vi "AssignFileChannels.vi"(10 "dataLoopCounter":dbl, 11 "dataTime_s":dbl) -> (3 "fileContent":T1)   [LabVIEW 2018]
uses:
  Clusters/FileDataChannel.ctl
  Clusters/IOSignals.ctl
  Clusters/ArrayPairs.ctl
  Clusters/SwapArrayCluster.ctl
  Clusters/GenCtrl.ctl
  Clusters/GenMode.ctl
  Clusters/PitchCtrl.ctl
  Clusters/BladePitchMode.ctl
  Clusters/RoscoParams.ctl
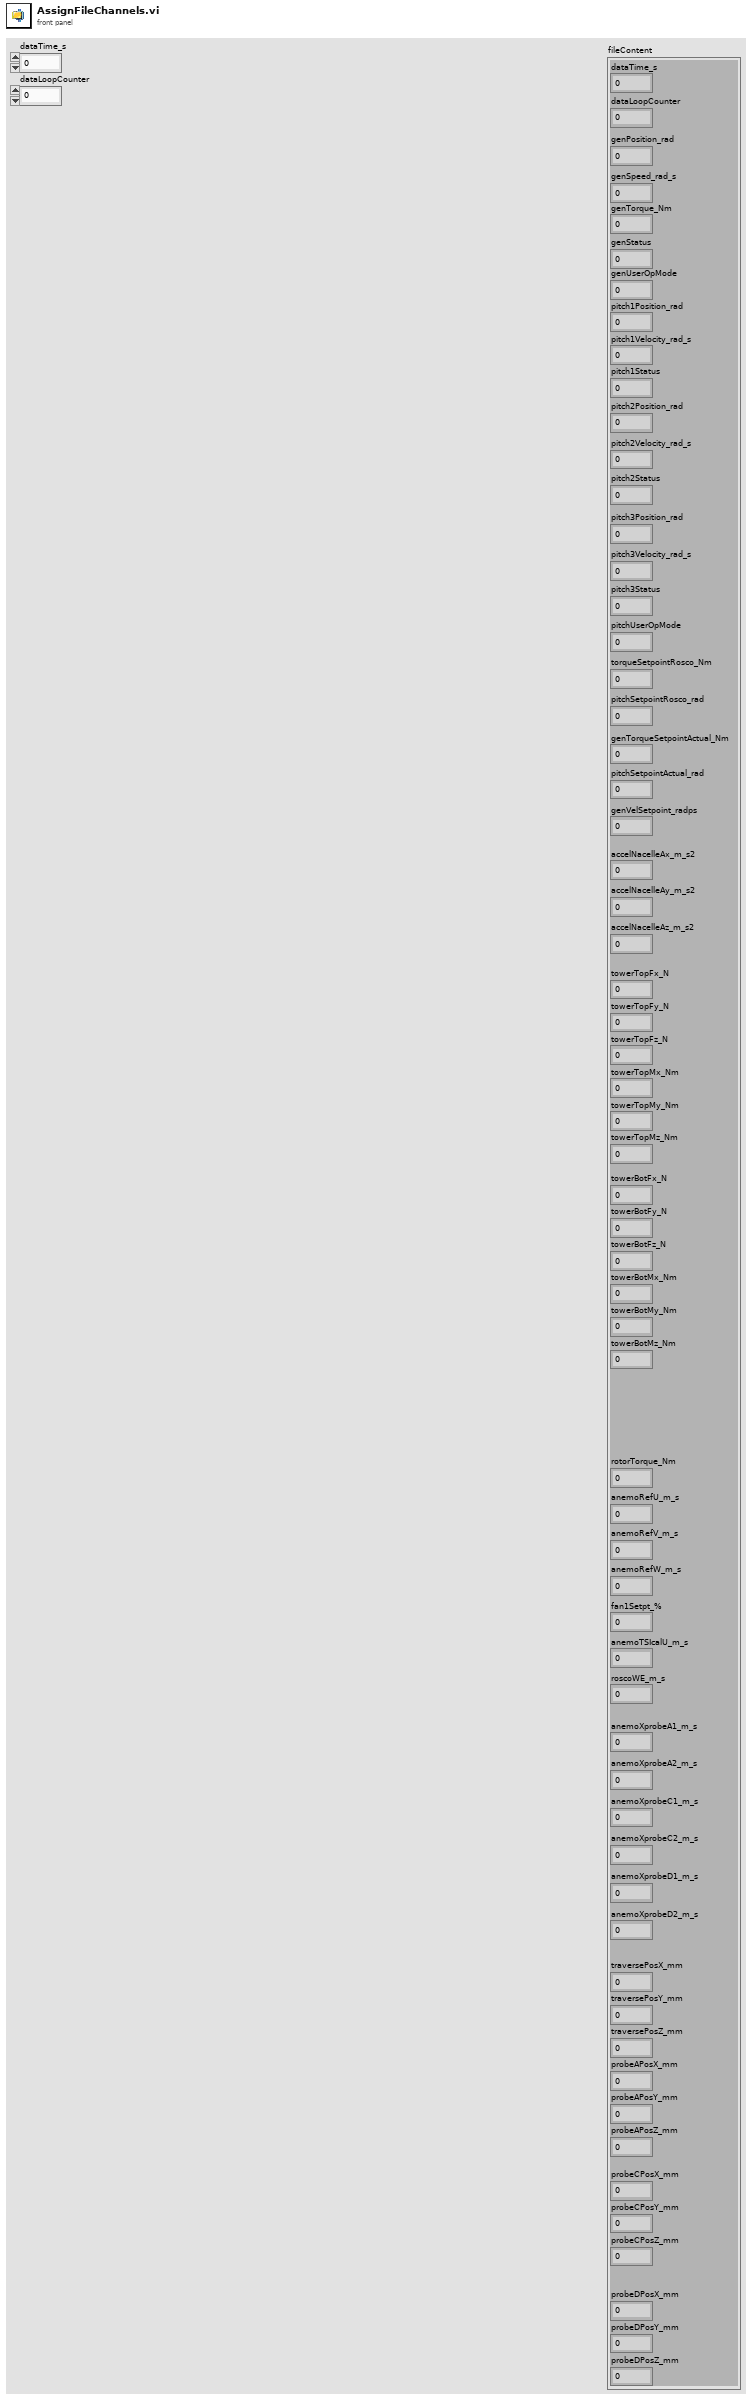
[diagram p1: front panel]
types:
  T1 = typedef "FileDataChannel.ctl" = cluster{"dataTime_s":dbl, "dataLoopCounter":dbl, "anemoRefU_m_s":dbl, "anemoRefV_m_s":dbl, "anemoRefW_m_s":dbl, "rotorTorque_Nm":dbl, "towerTopFx_N":dbl, "towerTopFy_N":dbl, "accelNacelleAx_m_s2":dbl, "accelNacelleAy_m_s2":dbl, "accelNacelleAz_m_s2":dbl, "genSpeed_rad_s":dbl, "genTorque_Nm":dbl, "genStatus":dbl, "pitch1Position_rad":dbl, "pitch1Velocity_rad_s":dbl, "pitch1Status":dbl, "pitch2Position_rad":dbl, "pitch2Velocity_rad_s":dbl, "pitch2Status":dbl, "pitch3Position_rad":dbl, "pitch3Velocity_rad_s":dbl, "pitch3Status":dbl, "genUserOpMode":dbl, "pitchUserOpMode":dbl, "torqueSetpointRosco_Nm":dbl, "pitchSetpointRosco_rad":dbl, "fan1Setpt_%":dbl, "genTorqueSetpointActual_Nm":dbl, "pitchSetpointActual_rad":dbl, "genVelSetpoint_radps":dbl, "genPosition_rad":dbl, "towerTopFz_N":dbl, "towerTopMx_Nm":dbl, "towerTopMy_Nm":dbl, "towerTopMz_Nm":dbl, "towerBotFx_N":dbl, "towerBotFy_N":dbl, "towerBotFz_N":dbl, "towerBotMx_Nm":dbl, "towerBotMy_Nm":dbl, "towerBotMz_Nm":dbl, "anemoTSIcalU_m_s":dbl, "roscoWE_m_s":dbl, "anemoXprobeA1_m_s":dbl, "anemoXprobeA2_m_s":dbl, "anemoXprobeC1_m_s":dbl, "anemoXprobeC2_m_s":dbl, "anemoXprobeD1_m_s":dbl, "anemoXprobeD2_m_s":dbl, "traversePosX_mm":dbl, "traversePosY_mm":dbl, "traversePosZ_mm":dbl, "probeAPosX_mm":dbl, "probeAPosY_mm":dbl, "probeAPosZ_mm":dbl, "probeCPosX_mm":dbl, "probeCPosY_mm":dbl, "probeCPosZ_mm":dbl, "probeDPosX_mm":dbl, "probeDPosY_mm":dbl, "probeDPosZ_mm":dbl}
  T2 = typedef "IOSignals.ctl" = cluster{"mainGenPosition (rad)":dbl, "mainGenVelocity (rad/s)":dbl, "motorCurrentTorq (Nm)":dbl, "mainGenStatus":u16, "pitch1Status":u16, "pitch1Position (rad)":dbl, "pitch1Velocity (rad/s)":dbl, "pitch1HomeFlag":bool, "pitch2Status":u16, "pitch2Position (rad)":dbl, "pitch2Velocity (rad/s)":dbl, "pitch2HomeFlag":bool, "pitch3Status":u16, "pitch3Position (rad)":dbl, "pitch3Velocity (rad/s)":dbl, "pitch3HomeFlag":bool, "torqueSensor (Nm)":dbl, "nacelleAccX (m/s2)":dbl, "nacelleAccY (m/s2)":dbl, "nacelleAccZ (m/s2)":dbl, "atiTowerTopFx_N":dbl, "atiTowerTopFy_N":dbl, "atiTowerTopFz_N":dbl, "atiTowerTopMx_Nm":dbl, "atiTowerTopMy_Nm":dbl, "atiTowerTopMz_Nm":dbl, "atiTowerBotFx_N":dbl, "atiTowerBotFy_N":dbl, "atiTowerBotFz_N":dbl, "atiTowerBotMx_Nm":dbl, "atiTowerBotMy_Nm":dbl, "atiTowerBotMz_Nm":dbl, "anemoRefU_m_s":dbl, "anemoRefV_m_s":dbl, "anemoRefW_m_s":dbl, "anemoCalU_m_s":dbl, "anemoXprobeA1_m_s":dbl, "anemoXprobeA2_m_s":dbl, "anemoXprobeC1_m_s":dbl, "anemoXprobeC2_m_s":dbl, "anemoXprobeD1_m_s":dbl, "anemoXprobeD2_m_s":dbl}
  T3 = typedef "GenCtrl.ctl" = cluster{"Constant velocity setpoint (rpm)":dbl, "Ramp target velocity (rpm)":dbl, "Ramp time (s)":dbl, "Sine mean (Nm)":dbl, "Sine amp (Nm)":dbl, "Sine period (s)":dbl, "Torque Ctrl I-Gain":dbl, "Velocity Ctrl P-Gain":dbl, "Velocity Ctrl I-Gain":dbl, "Max Torque (Nm)":dbl, "GeneratorOn":bool, "Torque Ctrl P-Gain":dbl, "From file velocity (rpm)":dbl, "Generator operating mode":T4, "Max Vel (rpm)":dbl, "Torque Ctrl FF Gain":dbl}
  T4 = typedef "GenMode.ctl" = enum32{"Velocity: Zero", "Velocity: Const.", "Velocity: Ramp", "Velocity: From File", "Torque: Sine", "Torque: ROSCO"}
  T5 = typedef "PitchCtrl.ctl" = cluster{"P-Gain":dbl, "Blade pitch operating mode":T6, "Constant setpoint (deg)":dbl, "I-Gain":dbl, "Pitch from File (deg)":dbl, "Homing vel (rpm)":dbl, "Max vel (rpm)":dbl, "Max vel change (rpm/min)":dbl}
  T6 = typedef "BladePitchMode.ctl" = enum32{"Zero pitch", "Const pitch", "From File", "ROSCO Ctrl"}
  T7 = typedef "ArrayPairs.ctl" = cluster{"iStatus":T8, "TIME":T8, "DT":T8, "Blade1PitchPos_rad":T8, "VS_MECHGENPWR":T8, "VS_GENPWR":T8, "GEN_SPEED":T8, "ROTOR_SPEED":T8, "GENTQMEAS":T8, "Y_M":T8, "HORWINDV":T8, "ROOTMOOP1":T8, "ROOTMOOP2":T8, "Blade2PitchPos_rad":T8, "Blade3PitchPos_rad":T8, "ROOTMOOP3":T8, "AVCMSG_SIZE":T8, "INFILE_SIZE ":T8, "OUTFILE_SIZE ":T8, "FA_ACC":T8, "NUM_BLADES":T8, "BladePitchSetpoint_rad":T8, "TorqueSetpoint_Nm":T8, "OUT_AEROTQ":T8, "Out.RotSpeed ":T8, "Out.DEBUG":T8}
  T8 = typedef "SwapArrayCluster.ctl" = cluster{"Index":i32, "Value":dbl}
  T9 = typedef "RoscoParams.ctl" = cluster{"avrSWAP":dbl[], "aviFAIL":i32, "currentMsg":string, "ReturnValue":i32, "disconInFileName":string, "outFileName":string, "firstMsg":string}
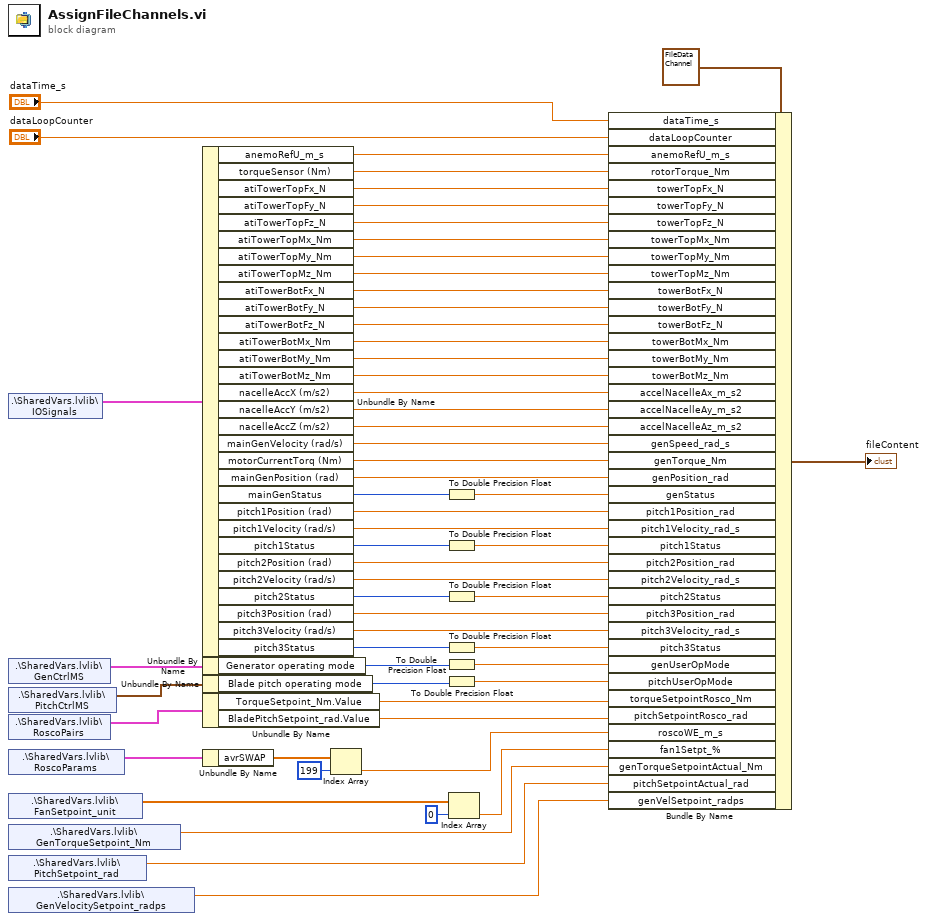
[diagram p0: block diagram]
diagram:
  n1 = shared-variable ".\\SharedVars.lvlib\\IOSignals"() -> (w57:T2)  [unwired: 1 in, 1 out]
  n2 = shared-variable ".\\SharedVars.lvlib\\GenCtrlMS"() -> (w39:T3)  [unwired: 1 in, 1 out]
  n3 = shared-variable ".\\SharedVars.lvlib\\PitchCtrlMS"() -> (w38:T5)  [unwired: 1 in, 1 out]
  n4 = shared-variable ".\\SharedVars.lvlib\\RoscoPairs"() -> (w40:T7)  [unwired: 1 in, 1 out]
  n5 = shared-variable ".\\SharedVars.lvlib\\RoscoParams"() -> (w11:T9)  [unwired: 1 in, 1 out]
  n6 = shared-variable ".\\SharedVars.lvlib\\FanSetpoint_unit"() -> (w25:dbl[])  [unwired: 1 in, 1 out]
  n7 = shared-variable ".\\SharedVars.lvlib\\GenTorqueSetpoint_Nm"() -> (w31:dbl)  [unwired: 1 in, 1 out]
  n8 = shared-variable ".\\SharedVars.lvlib\\PitchSetpoint_rad"() -> (w30:dbl)  [unwired: 1 in, 1 out]
  n9 = shared-variable ".\\SharedVars.lvlib\\GenVelocitySetpoint_radps"() -> (w29:dbl)  [unwired: 1 in, 1 out]
  n10 = Unbundle By Name(w57) -> ("anemoRefU_m_s"=w22:dbl, "torqueSensor (Nm)"=w23:dbl, "atiTowerTopFx_N"=w27:dbl, "atiTowerTopFy_N"=w26:dbl, "atiTowerTopFz_N"=w20:dbl, "atiTowerTopMx_Nm"=w18:dbl, "atiTowerTopMy_Nm"=w17:dbl, "atiTowerTopMz_Nm"=w16:dbl, "atiTowerBotFx_N"=w19:dbl, "atiTowerBotFy_N"=w5:dbl, "atiTowerBotFz_N"=w4:dbl, "atiTowerBotMx_Nm"=w3:dbl, "atiTowerBotMy_Nm"=w2:dbl, "atiTowerBotMz_Nm"=w1:dbl, "nacelleAccX (m/s2)"=w15:dbl, "nacelleAccY (m/s2)"=w14:dbl, "nacelleAccZ (m/s2)"=w13:dbl, "mainGenVelocity (rad/s)"=w56:dbl, "motorCurrentTorq (Nm)"=w55:dbl, "mainGenPosition (rad)"=w21:dbl, "mainGenStatus"=w53:u16, "pitch1Position (rad)"=w52:dbl, "pitch1Velocity (rad/s)"=w51:dbl, "pitch1Status"=w49:u16, "pitch2Position (rad)"=w48:dbl, "pitch2Velocity (rad/s)"=w47:dbl, "pitch2Status"=w46:u16, "pitch3Position (rad)"=w44:dbl, "pitch3Velocity (rad/s)"=w43:dbl, "pitch3Status"=w42:u16)
  n11 = Unbundle By Name(w39) -> ("Generator operating mode"=w37:T4)
  n12 = Unbundle By Name(w38) -> ("Blade pitch operating mode"=w34:T6)
  n13 = Unbundle By Name(w40) -> ("TorqueSetpoint_Nm.Value"=w33:dbl, "BladePitchSetpoint_rad.Value"=w32:dbl)
  n14 = Unbundle By Name(w11) -> ("avrSWAP"=w10:dbl[])
  n15 = Index Array(array=w10, index=199) -> (element=w8:dbl)
  n16 = To Double Precision Float(number=w53) -> (double precision float=w54:dbl)
  n17 = To Double Precision Float(number=w49) -> (double precision float=w50:dbl)
  n18 = To Double Precision Float(number=w46) -> (double precision float=w45:dbl)
  n19 = To Double Precision Float(number=w42) -> (double precision float=w41:dbl)
  n20 = To Double Precision Float(number=w37) -> (double precision float=w36:dbl)
  n21 = To Double Precision Float(number=w34) -> (double precision float=w35:dbl)
  n22 = Index Array(array=w25, index=0) -> (element=w9:dbl)
  n23 = Bundle By Name(cluster=T1 {"dataTime_s"=0.0, "dataLoopCounter"=0.0, "anemoRefU_m_s"=0.0, "anemoRefV_m_s"=0.0, "anemoRefW_m_s"=0.0, "rotorTorque_Nm"=0.0, "towerTopFx_N"=0.0, "towerTopFy_N"=0.0, "accelNacelleAx_m_s2"=0.0, "accelNacelleAy_m_s2"=0.0, "accelNacelleAz_m_s2"=0.0, "genSpeed_rad_s"=0.0, "genTorque_Nm"=0.0, "genStatus"=0.0, "pitch1Position_rad"=0.0, "pitch1Velocity_rad_s"=0.0, "pitch1Status"=0.0, "pitch2Position_rad"=0.0, "pitch2Velocity_rad_s"=0.0, "pitch2Status"=0.0, "pitch3Position_rad"=0.0, "pitch3Velocity_rad_s"=0.0, "pitch3Status"=0.0, "genUserOpMode"=0.0, "pitchUserOpMode"=0.0, "torqueSetpointRosco_Nm"=0.0, "pitchSetpointRosco_rad"=0.0, "fan1Setpt_%"=0.0, "genTorqueSetpointActual_Nm"=0.0, "pitchSetpointActual_rad"=0.0, "genVelSetpoint_radps"=0.0, "genPosition_rad"=0.0, "towerTopFz_N"=0.0, "towerTopMx_Nm"=0.0, "towerTopMy_Nm"=0.0, "towerTopMz_Nm"=0.0, "towerBotFx_N"=0.0, "towerBotFy_N"=0.0, "towerBotFz_N"=0.0, "towerBotMx_Nm"=0.0, "towerBotMy_Nm"=0.0, "towerBotMz_Nm"=0.0, "anemoTSIcalU_m_s"=0.0, "roscoWE_m_s"=0.0, "anemoXprobeA1_m_s"=0.0, "anemoXprobeA2_m_s"=0.0, "anemoXprobeC1_m_s"=0.0, "anemoXprobeC2_m_s"=0.0, "anemoXprobeD1_m_s"=0.0, "anemoXprobeD2_m_s"=0.0, "traversePosX_mm"=0.0, "traversePosY_mm"=0.0, "traversePosZ_mm"=0.0, "probeAPosX_mm"=0.0, "probeAPosY_mm"=0.0, "probeAPosZ_mm"=0.0, "probeCPosX_mm"=0.0, "probeCPosY_mm"=0.0, "probeCPosZ_mm"=0.0, "probeDPosX_mm"=0.0, "probeDPosY_mm"=0.0, "probeDPosZ_mm"=0.0} ("SwapIn"), "dataTime_s"="dataTime_s", "dataLoopCounter"="dataLoopCounter", "anemoRefU_m_s"=w22, "rotorTorque_Nm"=w23, "towerTopFx_N"=w27, "towerTopFy_N"=w26, "towerTopFz_N"=w20, "towerTopMx_Nm"=w18, "towerTopMy_Nm"=w17, "towerTopMz_Nm"=w16, "towerBotFx_N"=w19, "towerBotFy_N"=w5, "towerBotFz_N"=w4, "towerBotMx_Nm"=w3, "towerBotMy_Nm"=w2, "towerBotMz_Nm"=w1, "accelNacelleAx_m_s2"=w15, "accelNacelleAy_m_s2"=w14, "accelNacelleAz_m_s2"=w13, "genSpeed_rad_s"=w56, "genTorque_Nm"=w55, "genPosition_rad"=w21, "genStatus"=w54, "pitch1Position_rad"=w52, "pitch1Velocity_rad_s"=w51, "pitch1Status"=w50, "pitch2Position_rad"=w48, "pitch2Velocity_rad_s"=w47, "pitch2Status"=w45, "pitch3Position_rad"=w44, "pitch3Velocity_rad_s"=w43, "pitch3Status"=w41, "genUserOpMode"=w36, "pitchUserOpMode"=w35, "torqueSetpointRosco_Nm"=w33, "pitchSetpointRosco_rad"=w32, "roscoWE_m_s"=w8, "fan1Setpt_%"=w9, "genTorqueSetpointActual_Nm"=w31, "pitchSetpointActual_rad"=w30, "genVelSetpoint_radps"=w29) -> (→"fileContent":T1)
